vi "RSZVB Set Simultaneous Measurement Minimum Frequency Offset Mode.vi"(8 "error in (no error)":errorcluster {"code" format="%.0x"}, 9 "Minimum Frequency Offset (Bandwidth)":i32(ring)=1 items=["Direct", "Bandwidth"], 10 "Channel (1)":i32=1, 11 "VISA resource name":refnum<visa-resource-name>) -> (0 "error out":errorcluster {"code" format="%.0x"}, 3 "VISA resource name out":refnum<visa-resource-name>)   [LabVIEW 2011]
doc: "This VI defines how the minimum frequency offset between different port groups is determined for Simultaneous Measurement with Frequency Offset.\n\nRemote-control command(s):\nSOURce<Ch>:GROup:SIMultaneous:FOFFset:MOFFset:MODE DIRect | BANDwidth"
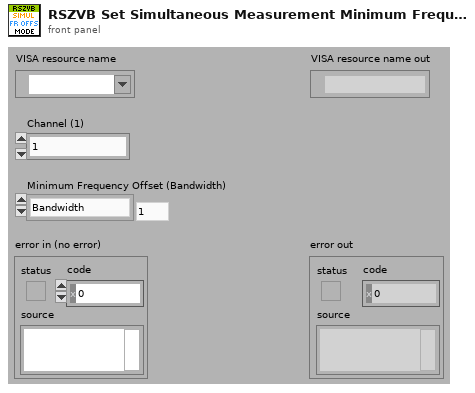
[diagram p1: front panel]
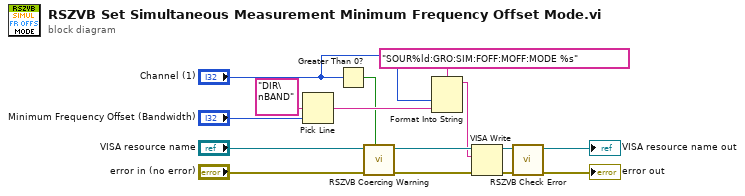
[diagram p0: block diagram]
diagram:
  n1 = Pick Line(multi-line string="DIR\nBAND", line index="Minimum Frequency Offset (Bandwidth)") -> (output string=w13:string)  [unwired: 1 in]
  n2 = Greater Than 0?(x="Channel (1)") -> (x > 0?=w11:bool)
  n3 = call "RSZVB Coercing Warning.vi"("In Range?"=w11, "error in (no error)"="error in (no error)", "VISA session"="VISA resource name") -> ("error out"=w12:errorcluster, "dup VISA session"=w10:refnum<visa-resource-name>)  [unwired: 7 in]
  n4 = Format Into String(format string="SOUR%ld:GRO:SIM:FOFF:MOFF:MODE %s", "Channel (1)", w13) -> (resulting string=w7:string)  [unwired: 2 in, 1 out]
  n5 = VISA Write(VISA resource name=w10, write buffer=w7, error in (no error)=w12) -> (VISA resource name out=w9:refnum<visa-resource-name>, error out=w8:errorcluster)  [unwired: 1 out]
  n6 = call "RSZVB Check Error.vi"("error in (no error)"=w8, "VISA session"=w9) -> ("error out"=→"error out":errorcluster, "dup VISA session"=→"VISA resource name out":refnum<visa-resource-name>)  [unwired: 8 in]
